vi "FTW-TransferClient-Destroy.vi"(0 "Transfer Client":refnum<class "FTW-TransferClient-S3.lvclass">, 11 "error in":errorcluster) -> (15 "error out":errorcluster)   [LabVIEW 2013, in "FTW-TransferClient-S3.lvclass"]
uses:
  FTW-TransferClient-S3.lvclass
  FTW-TransferClient.lvclass
  C:/Users/Jack/repo/ftw-master/Windows/src/Transfer Client/S3/AWSSDK.dll
  AWSSDK.dll
panel:
  # "Inputs"
  # "Outputs"
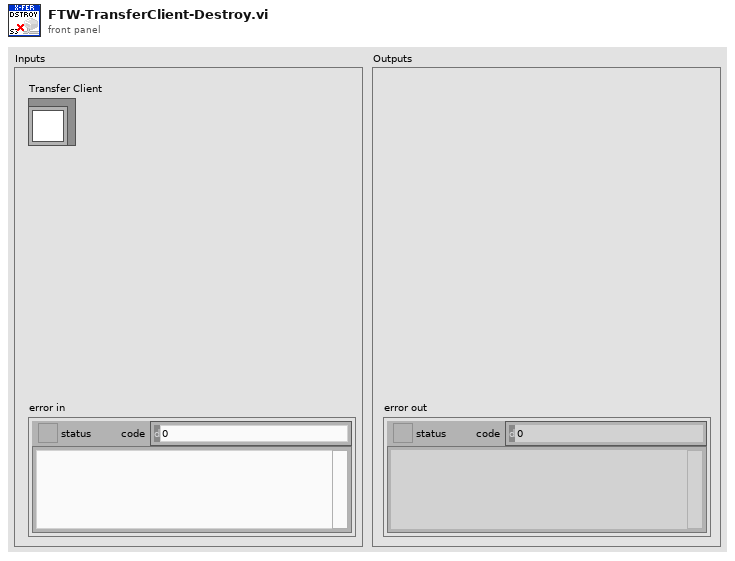
[diagram p1: front panel]
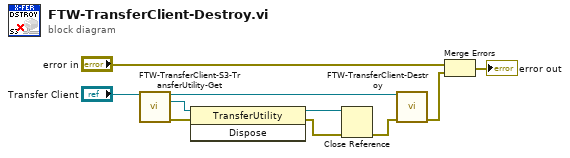
[diagram p0: block diagram]
diagram:
  n1 = call "FTW-TransferClient-S3-TransferUtility-Get.vi"("Transfer Client"="Transfer Client") -> ("Transfer Client out"=w9:refnum<class "FTW-TransferClient-S3.lvclass">, "Transfer Utility ref"=w8:refnum<k24>, "error out"=w7:errorcluster)  [unwired: 12 in]
  n2 = invoke class="TransferUtility" method="Dispose"(reference=w8, error in=w7) -> (reference out=w6:refnum<k24>, error out=w5:errorcluster)  [unwired: 1 in, 1 out]
  n3 = Close Reference(reference=w6, error in (no error)=w5) -> (error out=w4:errorcluster)
  n4 = call-parent "FTW-TransferClient-Destroy.vi"("Transfer Client"=w9, "error in"=w4) -> ("error out"=w1:errorcluster)  [unwired: 13 in]
  n5 = Merge Errors("error in", w1) -> (→"error out":errorcluster)
